vi "TDMS Advanced Synchronous Write.vi"   [LabVIEW 2023]
doc: "This example demonstrates how to write data synchronously to a .tdms file using the Advanced TDMS VIs and functions. You can use the TDMS Advanced Synchronous Read function to read data from the .tdms file."
uses:
  <vilib>/Utility/TDMS File Viewer/NI_TDMS File Viewer.lvlib
panel:
  # "Overview: Demonstrates the use of the Advanced TDMS functions to write a .tdms file synchronously.\nInstructions:\nRun this VI."
types:
  T1 = enum16{"open", "open or create", "create or replace", "create", "open (read-only)"}
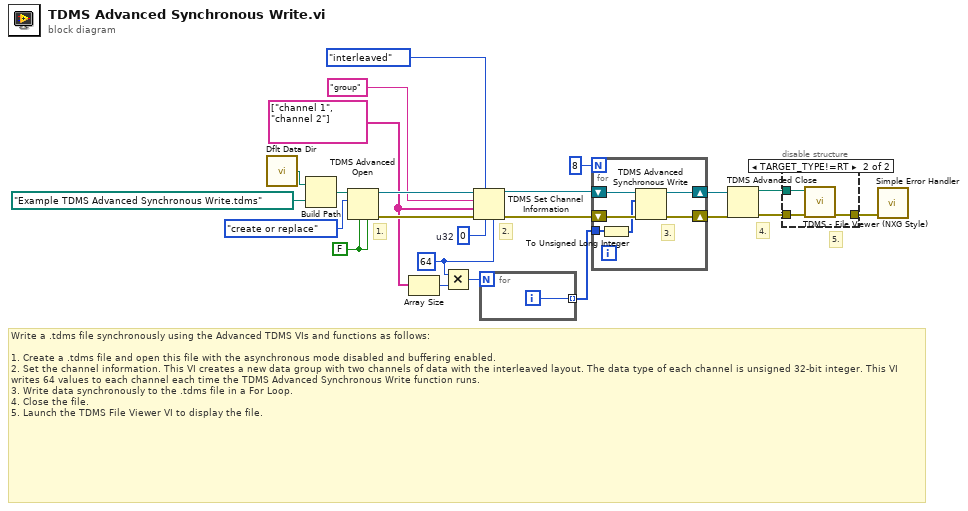
[diagram p0: block diagram]
diagram:
  w11 = FALSE ("enable asynchronous? (T)")
  w1 = u32 64 ("samples per channel")
  w12 = u32 0  # u32
  w2 = string[] ["channel 1", "channel 2"] ("channel name(s)")
  # "Write a .tdms file synchronously using the Advanced TDMS VIs and functions as follows:\n\n1. Create a .tdms file and open this file with the asynchronous mode disabled and buffering enabled.\n2. Set the channel information. This VI creates a new data group with two channels of data with the interleaved layout. The data type of each channel is unsigned 32-bit integer. This VI writes 64 values to each channel each time the TDMS Advanced Synchronous Write function runs.\n3. Write data synchronously to the .tdms file in a For Loop.\n4. Close the file.\n5. Launch the TDMS File Viewer VI to display the file."
  # "5."
  # "1."
  # "4."
  # "2."
  n1 = call <vilib>:"Dflt Data Dir.vi"() -> ("App:Default Data Directory"=w19:path)
  n2 = Build Path(base path=w19, name or relative path=path "Example TDMS Advanced Synchronous Write.tdms") -> (appended path=w23:path)
  n3 = TDMS Advanced Open(4:w11, 6:w11, 10:T1."create or replace" ("operation (0:open)"), 11:w23) -> (0:w21:errorcluster, 3:w20:refnum<k34>)  [unwired: 1 in, 1 out]
  n4 = Array Size(array=w2) -> (size(s)=w4:i32)
  n5 = Multiply(x=w1, y=w4) -> (x*y=w3:u32)
  n6 = TDMS Set Channel Information(4:w1, 6:w12, 7:enum16{"non-interleaved", "interleaved"}."interleaved" ("data layout (0:non-interleaved)"), 8:w21, 9:w2, 10:"group" ("group name (Untitled)"), 11:w20) -> (0:w10:errorcluster, 3:w9:refnum<k34>)
  n7 = for {
    N: w3 -> [_]
    tunnel: [w24] -> w15 mode=indexing
    i -> [w24]
  }
  n8 = for {
    N: 8 -> [_]
    shift-right: [w27] -> w13
    shift-left: w9 -> [w29]
    shift-right: [w28] -> w14
    shift-left: w10 -> [w30]
    tunnel: w15 -> [w26]
    # "3."
    n9 = To Unsigned Long Integer(number=w26) -> (unsigned 32bit integer=w25:u32[])
    n10 = TDMS Advanced Synchronous Write(8:w30, 10:w25, 11:w29) -> (0:w28:errorcluster, 3:w27:refnum<k34>)
  }
  n11 = TDMS Advanced Close(8:w14, 11:w13) -> (0:w6:errorcluster, 3:w7:path)  [unwired: 2 in]
  n12 = disable-structure shown="TARGET_TYPE!=RT" {
    disable-tunnel: w6 -> [w31 w34]
    disable-tunnel: w7 -> [_ w33]
    disable-tunnel: [w31 w32] -> w5
    frame condition #0 {
    }
    frame condition #1 (active) {
      n13 = call <vilib>:"TDMS - File Viewer (NXG Style).vi"("error in"=w34, "file in"=w33) -> ("error out"=w32:errorcluster)  [unwired: 8 in, 1 out]
    }
  }
  n14 = call <vilib>:"Simple Error Handler.vi"("error in (no error)"=w5) -> ()  [unwired: 4 in, 5 out]
